vi "LM model function and gradient_step.vi"(3 "output control":T1, 4 "data":variant, 5 "X":dbl[](array[numeric]), 6 "a":dbl[](array[numeric])) -> (0 "error out":errorcluster, 1 "f'(X,a)":dbl[][](array[numeric]), 2 "f(X,a)":dbl[](array[numeric]))   [LabVIEW 2016]
doc: "This template is the starting point for creating a model function to be passed to the Nonlinear Curve Fit.vi."
uses:
  <vilib>/gmath/NumericalOptimization/LM_output select.ctl
  <vilib>/gmath/NI_Gmath.lvlib
panel:
  out "loop":i32
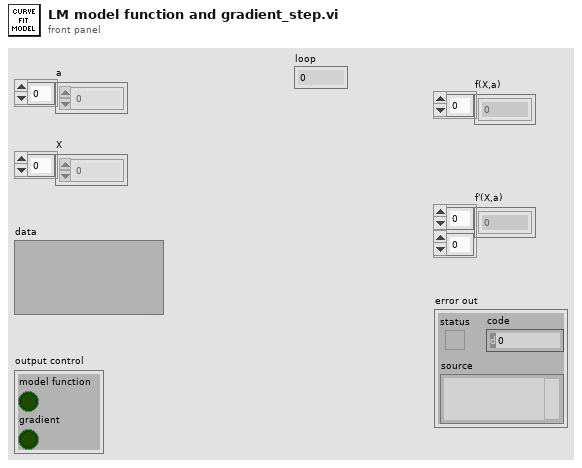
[diagram p1: front panel]
types:
  T1 = typedef "NI_Gmath.lvlib/LM_output select.ctl" = cluster{"model function":bool, "gradient":bool}
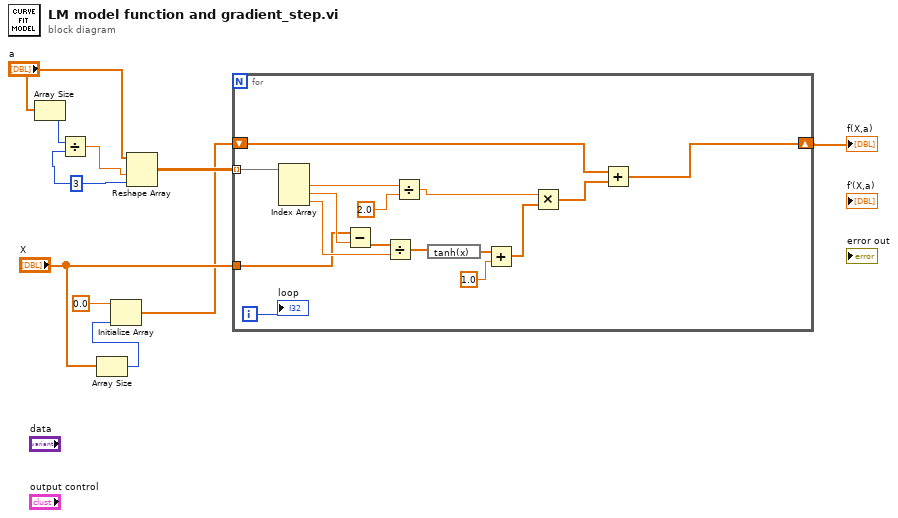
[diagram p0: block diagram]
diagram:
  w2 = 3 ("dimension size")
  n1 = Array Size(array="a") -> (size(s)=w3:i32)
  n2 = Divide(x=w3, y=w2) -> (x/y=w1:dbl)
  n3 = Array Size(array="X") -> (size(s)=w7:i32)
  n4 = Initialize Array(0.0 ("element"), w7) -> (w6:dbl[])
  n5 = Reshape Array("a", w1, w2) -> (w10:dbl[][])
  n6 = for {
    tunnel: w10 -> [w26] mode=indexing
    tunnel: "X" -> [w12]
    shift-right: [w14] -> w5
    shift-left: w6 -> [w15]
    i -> [w11]
    n7 = Index Array(array=w26) -> (element #1=w25:dbl, element #2=w13:dbl, element #3=w21:dbl)  [unwired: 3 in]
    n8 = Subtract(x=w12, y=w13) -> (x-y=w22:dbl[])
    n9 = Divide(x=w22, y=w21) -> (x/y=w20:dbl[])
    n10 = Divide(x=w25, y=2.0) -> (x/y=w23:dbl)
    n11 = expression code="tanh(x)"(w20) -> (w19:dbl[])
    n12 = Add(x=w19, y=1.0) -> (x+y=w17:dbl[])
    n13 = Multiply(x=w23, y=w17) -> (x*y=w16:dbl[])
    n14 = Add(x=w15, y=w16) -> (x+y=w14:dbl[])
    "loop" <- w11
  }
  "f(X,a)" <- w5
